vi "Facade.vi"(0 "Data In":T4, 2 "Display State In":T2, 3 "Container State":T3) -> (6 "Data Out":T4, 7 "Display State Out":T2, 8 "Action":T1)   [LabVIEW 2012, in "String XControl.xctl"]
uses:
  String XControl.xctl
  Data.ctl
  <vilib>/_xctls/Container State.ctl
  State.ctl
  <vilib>/_xctls/Action.ctl
  <vilib>/_xctls/XControlSupport.lvlib
panel:
  out "2D Picture":picture
types:
  T1 = typedef "XControlSupport.lvlib/Action.ctl" = cluster{"Data Changed?":bool, "State Changed?":bool, "Action Name":string}
  T2 = typedef "String XControl.xctl/State.ctl" = cluster{"Autoscale Font Size?":bool, "Alignment":cluster{"horizontal":enum16{"left", "center", "right"}, "vertical":enum16{"top", "center", "bottom"}}, "Font":cluster{"Font Name:":string, "Size":i16, "Strikeout?":bool, "Italic?":bool, "Underline?":bool, "Outline?":bool, "Shadow?":bool, "Bold?":bool}, "Text Color":u32, "BG Color":u32}
  T3 = typedef "XControlSupport.lvlib/Container State.ctl" = cluster{"Indicator?":bool, "Run Mode?":bool, " Refnum":refnum<vi>}
  T4 = typedef "String XControl.xctl/Data.ctl" = string
  T5 = cluster{"horizontal":enum16{"left", "center", "right"}, "vertical":enum16{"top", "center", "bottom"}}
  T6 = cluster{"Font Name:":string, "Size":i16, "Strikeout?":bool, "Italic?":bool, "Underline?":bool, "Outline?":bool, "Shadow?":bool, "Bold?":bool}
  T7 = typedef "LVBoundsTypeDef.ctl" = cluster{"Width":u32, "Height":u32}
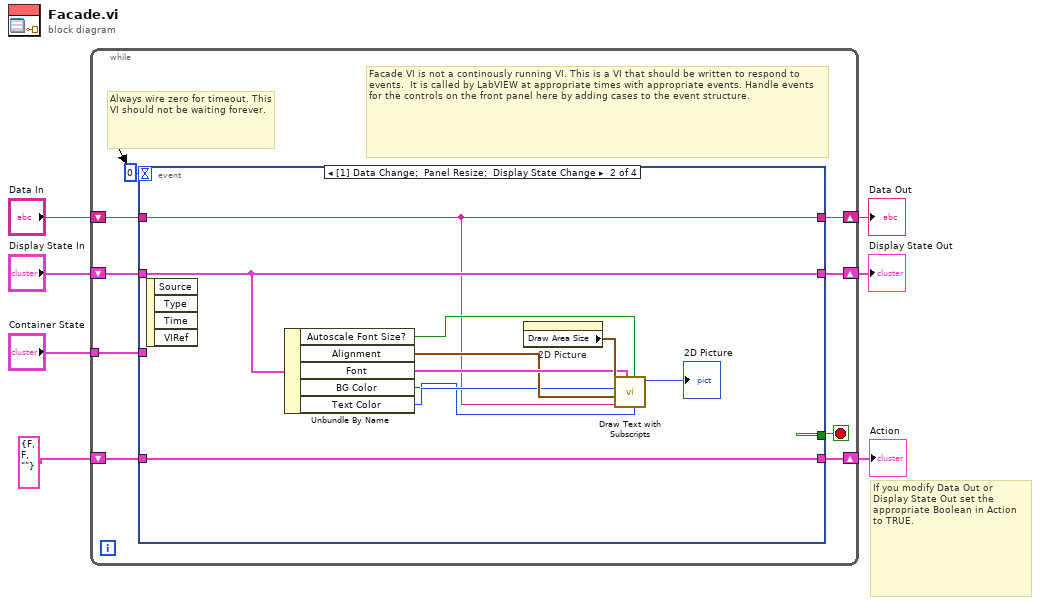
[diagram p0: block diagram]
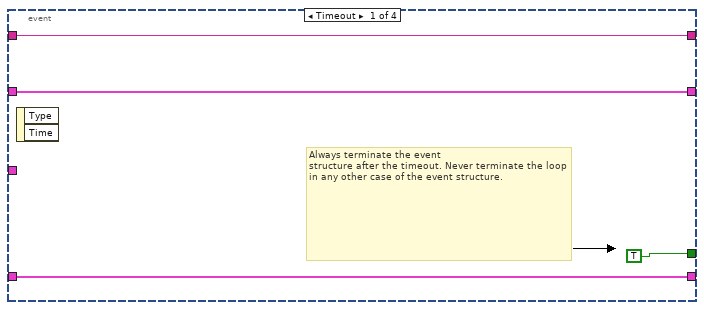
[diagram p2: hidden frame]
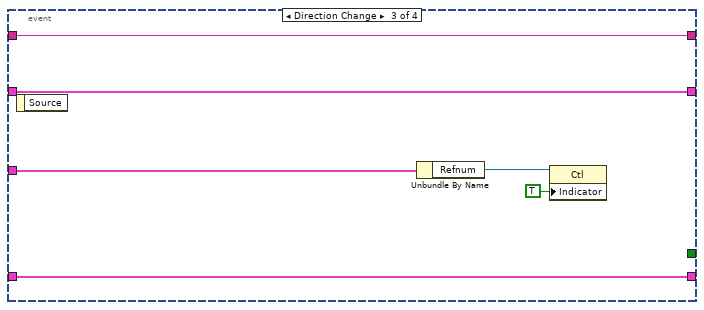
[diagram p3: hidden frame]
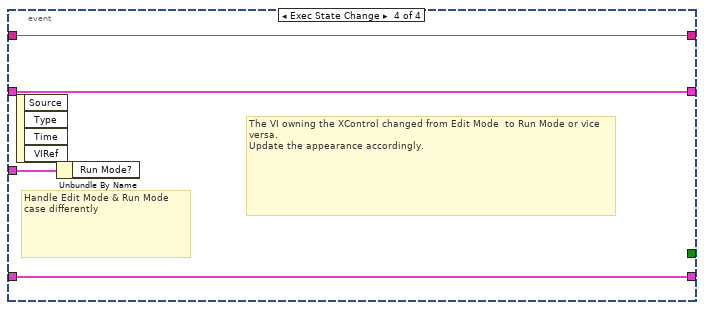
[diagram p4: hidden frame]
diagram:
  # "If you modify Data Out or\nDisplay State Out set the\nappropriate Boolean in Action\nto TRUE."
  n1 = while {
    shift-right: [w15] -> w4
    shift-left: "Display State In" -> [w16]
    tunnel: "Container State" -> [w12]
    shift-right: [w10] -> w7
    shift-left: "Data In" -> [w11]
    shift-right: [w8] -> w2
    shift-left: T1 {"Data Changed?"=FALSE, "State Changed?"=FALSE, "Action Name"=""} ("Action") -> [w9]
    stop <- w14 stop-if-true
    # "Facade VI is not a continously running VI. This is a VI that should be written to respond to events.  It is called by LabVIEW at appropriate times with appropriate events. Handle events for the controls on the front panel here by adding cases to the event structure."
    # "Always wire zero for timeout. This\nVI should not be waiting forever."
    n2 = event shown="[1] Data Change;  Panel Resize;  Display State Change" {
      selector: _ -> [_ _ _ _]
      dyn-events: _ -> [_ _ _ _]
      timeout: 0 -> [_ _ _ _]
      tunnel: w16 -> [w18 w27 w35 w39]
      tunnel: [w18 w27 w35 w39] -> w15
      tunnel: [TRUE _ _ _] -> w14
      tunnel: w12 -> [_ _ w36 w40]
      tunnel: w11 -> [w17 w21 w34 w38]
      tunnel: [w17 w21 w34 w38] -> w10
      tunnel: [w19 w30 w33 w37] -> w8
      tunnel: w9 -> [w19 w30 w33 w37]
      event Timeout {
        # "Always terminate the event\nstructure after the timeout. Never terminate the loop in any other case of the event structure."
        n3 = event-data() -> ()  [unwired: 1 in, 2 out]
      }
      event Data Change; Panel Resize; Display State Change {
        n4 = event-data() -> ()  [unwired: 1 in, 4 out]
        n5 = Unbundle By Name(w27) -> ("Autoscale Font Size?"=w25:bool, "Alignment"=w24:T5, "Font"=w26:T6, "BG Color"=w22:u32, "Text Color"=w23:u32)
        n6 = property on="2D Picture" class="Pict"() -> ("Draw Area Size"=w29:T7)  [unwired: 2 in, 2 out]
        n7 = call "Draw Text with Subscripts.vi"("BG color(transparent)"=w22, "Autoscale Font Size?"=w25, "Font"=w26, "String"=w21, "alignment(left, top)"=w24, "text color(black)"=w23, "Draw Area Size"=w29) -> ("new picture"=→"2D Picture":picture)  [unwired: 4 in]
      }
      event Direction Change {
        n8 = event-data() -> ()  [unwired: 1 in, 1 out]
        n9 = Unbundle By Name(w36) -> ("Refnum"=w32:refnum<vi>)
        n10 = property class="Ctl"(reference=w32, "Indicator"=TRUE) -> ()  [unwired: 1 in, 2 out]
      }
      event Exec State Change {
        # "The VI owning the XControl changed from Edit Mode  to Run Mode or vice versa.\nUpdate the appearance accordingly."
        # "Handle Edit Mode & Run Mode\ncase differently"
        n11 = event-data() -> ()  [unwired: 1 in, 4 out]
        n12 = Unbundle By Name(w40) -> ()  [unwired: 1 out]
      }
    }
  }
  "Display State Out" <- w4
  "Data Out" <- w7
  "Action" <- w2
